vi "filter.hostToFpga.testRunner.vi"(6 "Request.Debug?":bool, 8 "error in":errorcluster, 9 "Watch.List":string[](array[string])=["AAPL"], 10 "Expected OrderBook.Command[]":T1[](array[typedef])=[{"OrderBook Command.Type"=enum."AddOrder", "Side (U8)"=66, "Order Id (U64)"=3544385890602799695, "Quantity (U32)"=20000, "Symbol (U64)"=4702127773838213120, "Price (U64)"=9050, "Executed Quantity (U32)"=0, "Canceled Quantity (U32)"=0, "Remaining Quantity (U32)"=0, "Seconds (U64)"=0, "Nanoseconds (U64)"=0}, {"OrderBook Command.Type"=enum."AddOrder", "Side (U8)"=66, "Order Id (U64)"=3616443484640727631, "Quantity (U32)"=20000, "Symbol (U64)"=4702127773838213120, "Price (U64)"=9050, "Executed Quantity (U32)"=0, "Canceled Quantity (U32)"=0, "Remaining Quantity (U32)"=0, "Seconds (U64)"=0, "Nanoseconds (U64)"=0}, {"OrderBook Command.Type"=enum."AddOrder", "Side (U8)"=66, "Order Id (U64)"=3688501078678655567, "Quantity (U32)"=20000, "Symbol (U64)"=4702127773838213120, "Price (U64)"=9050, "Executed Quantity (U32)"=0, "Canceled Quantity (U32)"=0, "Remaining Quantity (U32)"=0, "Seconds (U64)"=0, "Nanoseconds (U64)"=0}, {"OrderBook Command.Type"=enum."AddOrder", "Side (U8)"=66, "Order Id (U64)"=3760558672716583503, "Quantity (U32)"=20000, "Symbol (U64)"=4702127773838213120, "Price (U64)"=9050, "Executed Quantity (U32)"=0, "Canceled Quantity (U32)"=0, "Remaining Quantity (U32)"=0, "Seconds (U64)"=0, "Nanoseconds (U64)"=0}, {"OrderBook Command.Type"=enum."AddOrder", "Side (U8)"=66, "Order Id (U64)"=3832616266754511439, "Quantity (U32)"=20000, "Symbol (U64)"=4702127773838213120, "Price (U64)"=9050, "Executed Quantity (U32)"=0, "Canceled Quantity (U32)"=0, "Remaining Quantity (U32)"=0, "Seconds (U64)"=0, "Nanoseconds (U64)"=0}, {"OrderBook Command.Type"=enum."AddOrder", "Side (U8)"=66, "Order Id (U64)"=3904673860792439375, "Quantity (U32)"=20000, "Symbol (U64)"=4702127773838213120, "Price (U64)"=9050, "Executed Quantity (U32)"=0, "Canceled Quantity (U32)"=0, "Remaining Quantity (U32)"=0, "Seconds (U64)"=0, "Nanoseconds (U64)"=0}, {"OrderBook Command.Type"=enum."AddOrder", "Side (U8)"=66, "Order Id (U64)"=3976731454830367311, "Quantity (U32)"=20000, "Symbol (U64)"=4702127773838213120, "Price (U64)"=9050, "Executed Quantity (U32)"=0, "Canceled Quantity (U32)"=0, "Remaining Quantity (U32)"=0, "Seconds (U64)"=0, "Nanoseconds (U64)"=0}, {"OrderBook Command.Type"=enum."AddOrder", "Side (U8)"=66, "Order Id (U64)"=4048789048868295247, "Quantity (U32)"=20000, "Symbol (U64)"=4702127773838213120, "Price (U64)"=9050, "Executed Quantity (U32)"=0, "Canceled Quantity (U32)"=0, "Remaining Quantity (U32)"=0, "Seconds (U64)"=0, "Nanoseconds (U64)"=0}, {"OrderBook Command.Type"=enum."AddOrder", "Side (U8)"=66, "Order Id (U64)"=4120846642906223183, "Quantity (U32)"=20000, "Symbol (U64)"=4702127773838213120, "Price (U64)"=9050, "Executed Quantity (U32)"=0, "Canceled Quantity (U32)"=0, "Remaining Quantity (U32)"=0, "Seconds (U64)"=0, "Nanoseconds (U64)"=0}, {"OrderBook Command.Type"=enum."AddOrder", "Side (U8)"=66, "Order Id (U64)"=4697307395209646671, "Quantity (U32)"=20000, "Symbol (U64)"=4702127773838213120, "Price (U64)"=9050, "Executed Quantity (U32)"=0, "Canceled Quantity (U32)"=0, "Remaining Quantity (U32)"=0, "Seconds (U64)"=0, "Nanoseconds (U64)"=0}, {"OrderBook Command.Type"=enum."AddOrder", "Side (U8)"=66, "Order Id (U64)"=4769364989247574607, "Quantity (U32)"=20000, "Symbol (U64)"=4702127773838213120, "Price (U64)"=9050, "Executed Quantity (U32)"=0, "Canceled Quantity (U32)"=0, "Remaining Quantity (U32)"=0, "Seconds (U64)"=0, "Nanoseconds (U64)"=0}] {"Side (U8)" format="%.0x"; "Order Id (U64)" format="%.0x"; "Symbol (U64)" format="%.0x"}, 11 "OrderBook.Commands.in":T1[](array[typedef]) {"Side (U8)" format="%.0x"; "Order Id (U64)" format="%.0x"; "Symbol (U64)" format="%.0x"}) -> (0 "error out":errorcluster={"status"=TRUE, "code"=-61165, "source"="Open FPGA VI Reference in host.bats.parser.tester.vi"}, 1 "Failures.Count":i32, 2 "Passed":bool, 3 "OrderBook.Commands.out":T1[](array[typedef]) {"Side (U8)" format="%.0x"; "Order Id (U64)" format="%.0x"; "Symbol (U64)" format="%.0x"}, 4 "Debug":u64[](array[numeric]) format="%.0x", 5 "GetState":u64[](array[numeric]) format="%.0x")   [LabVIEW 2022 SP3]
uses:
  fpga/common/orderbook.command.ctl
  fpga/common/orderbook.command.type.ctl
  <vilib>/rvi/interface/RandomDataEmulation/nirviRandomDataOpen.vi
  <vilib>/rvi/interface/common/niFpgaCacheSessionInfoDynamic.vi
  <vilib>/Utility/error.llb/Error Cluster From Error Code.vi
  <vilib>/rvi/errors/niLvFpgaAdjustHostInterfaceError.vi
  <vilib>/FPGAPlugInAG/Dynamic/niLvFpga_Close_Dynamic.vi
  <vilib>/rvi/interface/nirviOpenFPGA/nirviOpenFPGA.xnode
  fpga/filter/filter.test.vi
  <vilib>/rvi/interface/nirviReadWriteControl/nirviReadWriteControl.xnode
  <vilib>/rvi/interface/nirviMethod/nirviMethod.xnode
  <vilib>/rvi/interface/nirviCloseFPGA/nirviCloseFPGA.xnode
  <vilib>/rvi/errors/niLvFpgaMergeErrorWithErrorCode.vi
  <vilib>/FPGAPlugInAG/Dynamic/niLvFpga_ReadFifo_Dynamic.vi
  <vilib>/rvi/interface/Simulation/niFpgaSimulationCallBeginRW.vi
  NiFpgaLv.dll
  <vilib>/FPGAPlugInAG/Dynamic/niLvFpga_WriteFifo_Dynamic.vi
panel:
  out "HT-Filter.Commands.In":u64[](array[numeric])=[1, 66, 48, 20000, 4702127773838221344, 9050, 0, 0, 0, 0, 0, 0, 0, 0, 0, 0, 2, 66, 48, 0, 0, 9050, 200, 0, 0, 0, 0, 0, 0, 0, 0, 0, 5, 66, 48, 1400, 6076284164848492576, 9050, 0, 0, 0, 0, 0, 0, 0, 0, 0, 0] format="%.0x"
  out "Failures.Details":bool[][](array[boolean])
  out "Data.size":i32
  in  "Execute?":bool=TRUE
  out "Data":u64[](array[numeric]) format="%.0x"
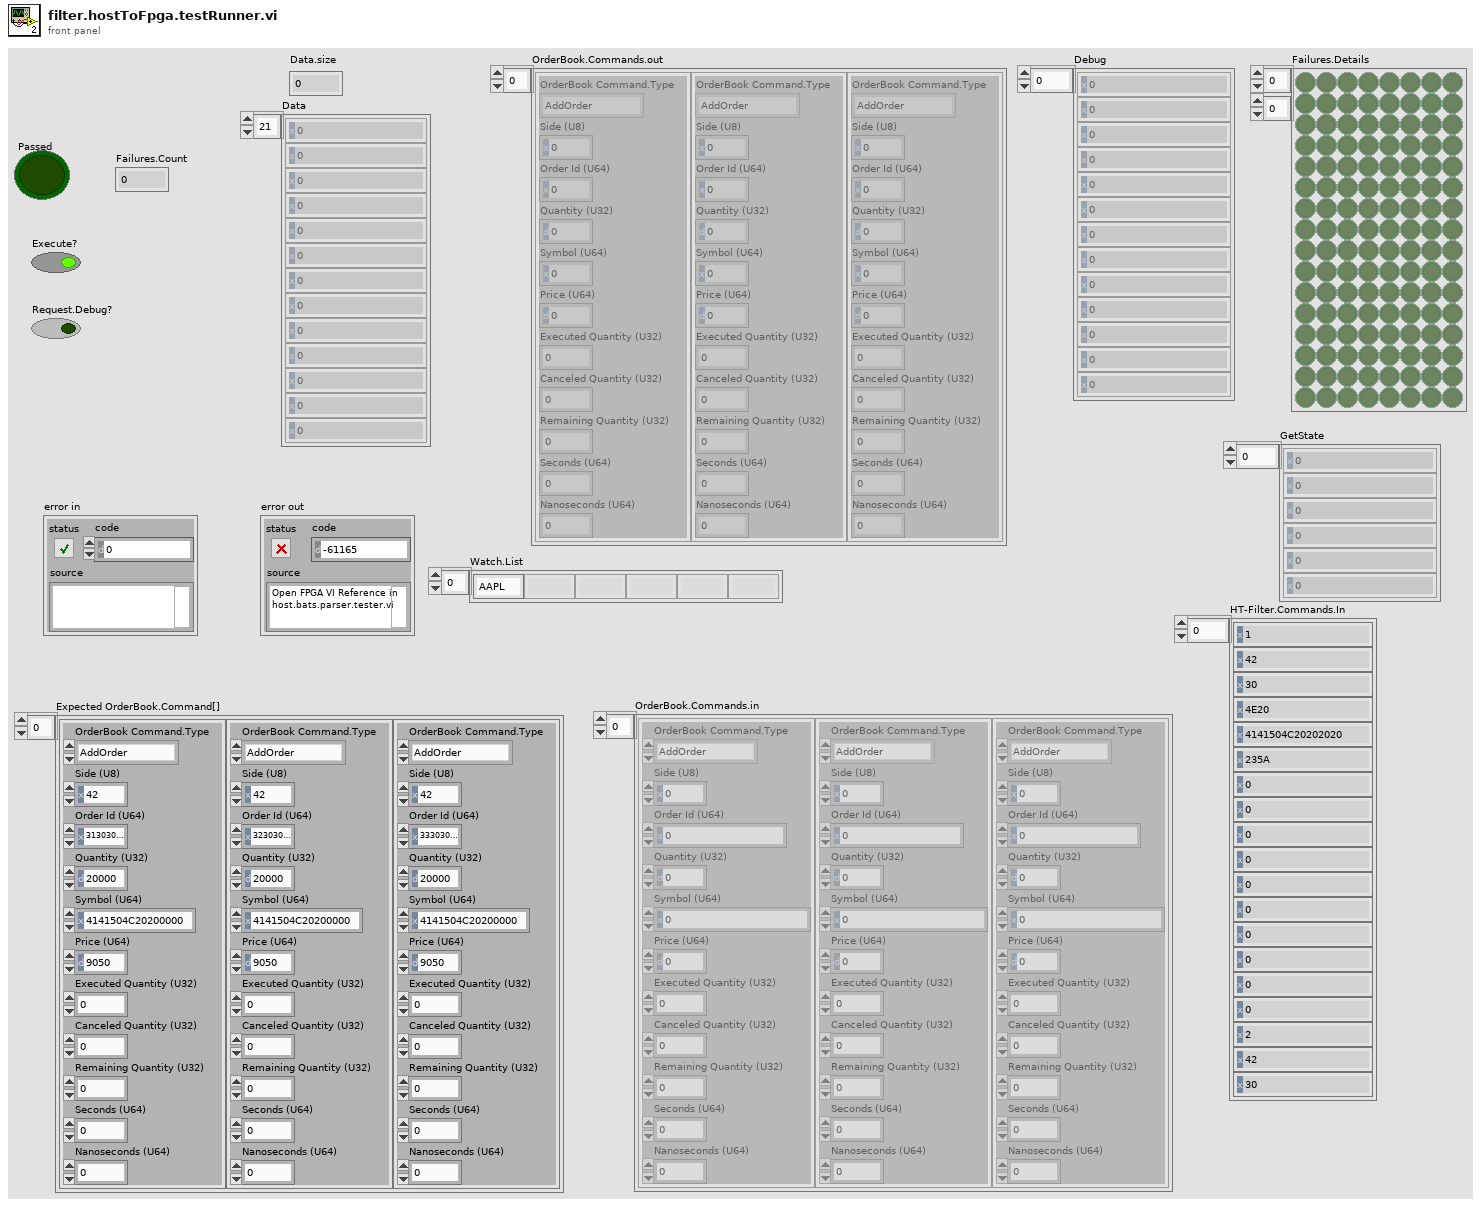
[diagram p1: front panel]
types:
  T1 = typedef "orderbook.command.ctl" = cluster{"OrderBook Command.Type":T2, "Side (U8)":u8, "Order Id (U64)":u64, "Quantity (U32)":u32, "Symbol (U64)":u64, "Price (U64)":u64, "Executed Quantity (U32)":u32, "Canceled Quantity (U32)":u32, "Remaining Quantity (U32)":u32, "Seconds (U64)":u64, "Nanoseconds (U64)":u64}
  T2 = typedef "orderbook.command.type.ctl" = enum16{"Time", "AddOrder", "OrderExecuted", "OrderExecutedAtPrice", "ReduceSize", "ModifyOrder", "DeleteOrder", "Get.State", "Get.All.Orders", "Get.Top"}
  T3 = cluster{"OrderBook Command.Type":bool, "Side (U8)":bool, "Order Id (U64)":bool, "Quantity (U32)":bool, "Symbol (U64)":bool, "Price (U64)":bool, "Executed Quantity (U32)":bool, "Cancelled Quantity (U32)":bool, "Cancelled Quantity (U32) 2":bool, "Executed Quantity (U32) 2":bool, "Cancelled Quantity (U32) 3":bool}
  T4 = cluster{"Index":i32, "x = y?":cluster{"OrderBook Command.Type":bool, "Side (U8)":bool, "Order Id (U64)":bool, "Quantity (U32)":bool, "Symbol (U64)":bool, "Price (U64)":bool, "Executed Quantity (U32)":bool, "Cancelled Quantity (U32)":bool, "Cancelled Quantity (U32) 2":bool, "Executed Quantity (U32) 2":bool, "Cancelled Quantity (U32) 3":bool}}
  T5 = cluster{"Index":i32, "x = y?":cluster{"OrderBook Command.Type":bool, "Side (U8)":bool, "Order Id (U64)":bool, "Quantity (U32)":bool, "Symbol (U64)":bool, "Price (U64)":bool, "Executed Quantity (U32)":bool, "Cancelled Quantity (U32)":bool, "Cancelled Quantity (U32) 2":bool, "Executed Quantity (U32) 2":bool, "Cancelled Quantity (U32) 3":bool}}[]
  T6 = cluster{"OrderBook Command.Type":bool, "Side (U8)":bool, "Order Id (U64)":bool, "Quantity (U32)":bool, "Symbol (U64)":bool, "Price (U64)":bool, "Executed Quantity (U32)":bool, "Canceled Quantity (U32)":bool, "Remaining Quantity (U32)":bool, "Seconds (U64)":bool, "Nanoseconds (U64)":bool}
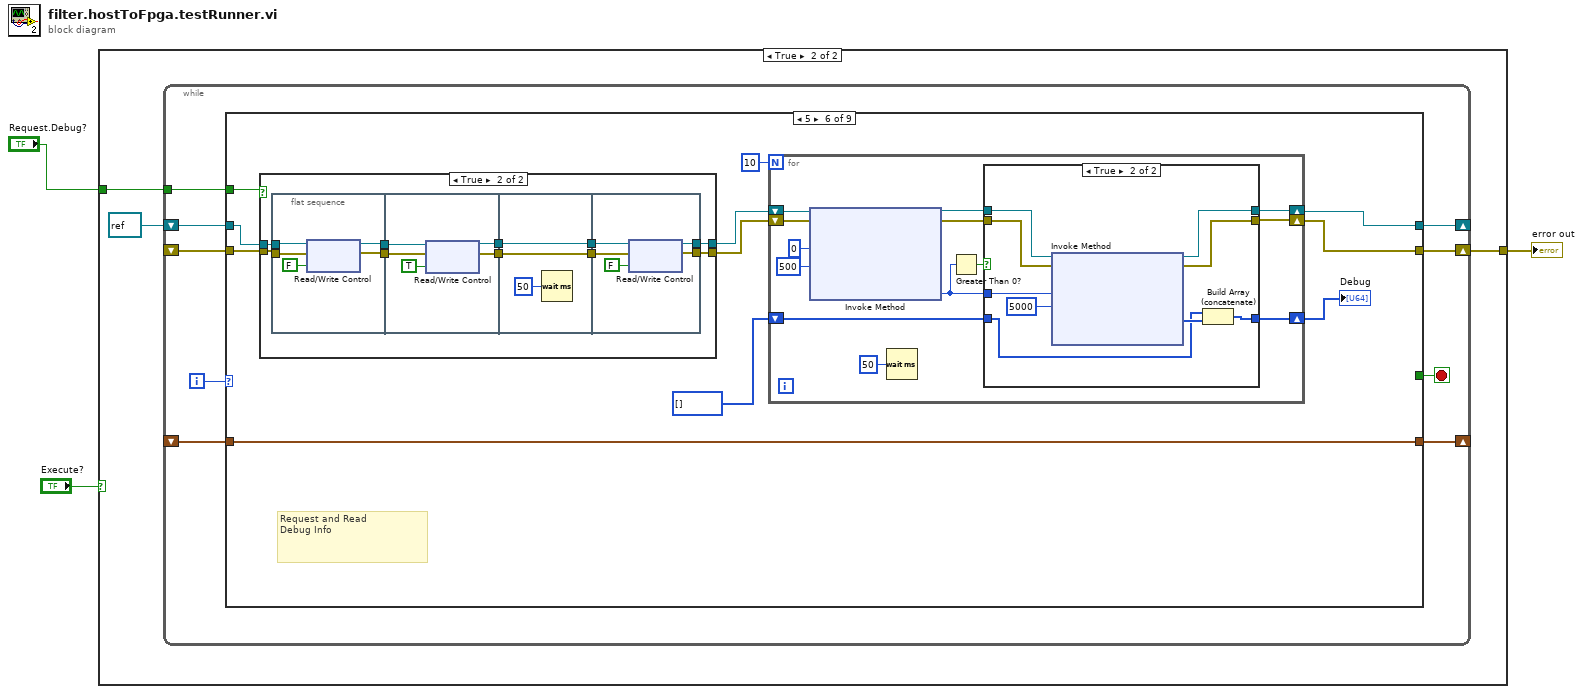
[diagram p0: block diagram]
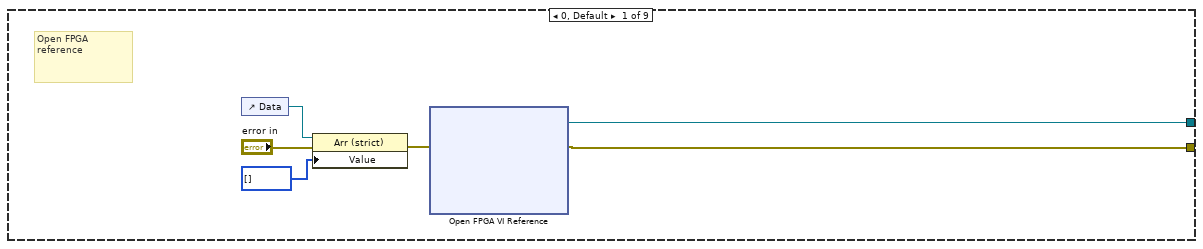
[diagram p3: hidden frame]
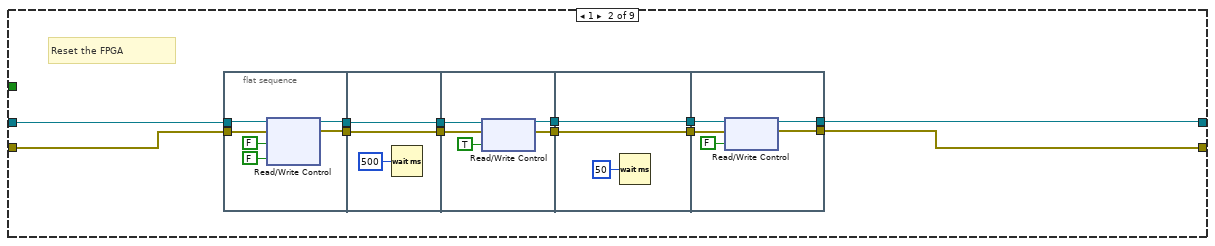
[diagram p4: hidden frame]
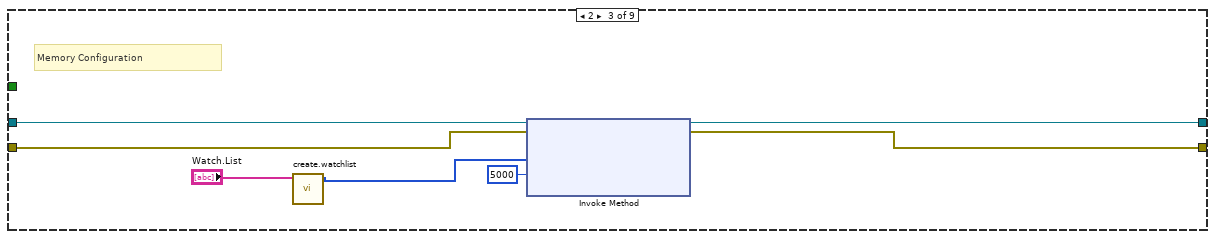
[diagram p5: hidden frame]
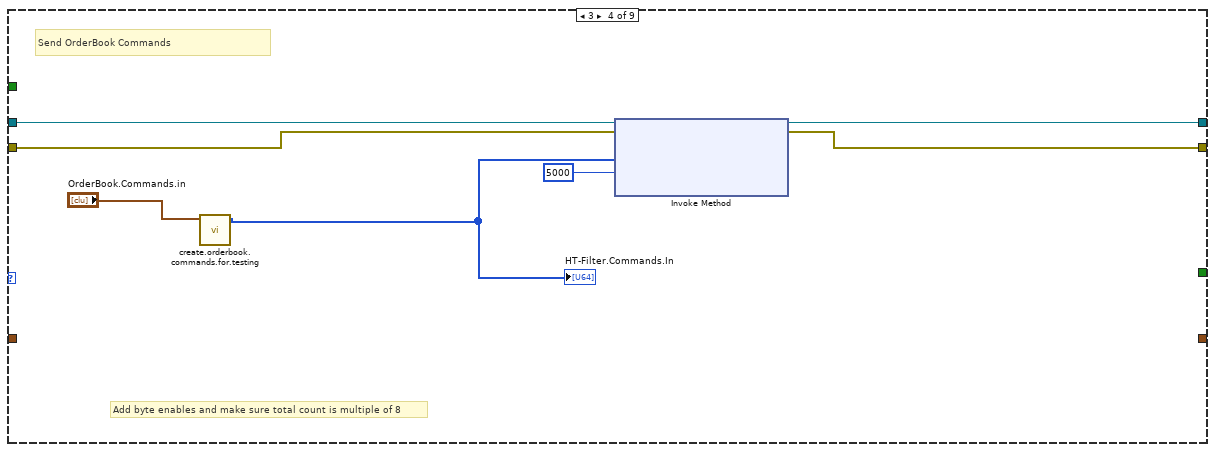
[diagram p6: hidden frame]
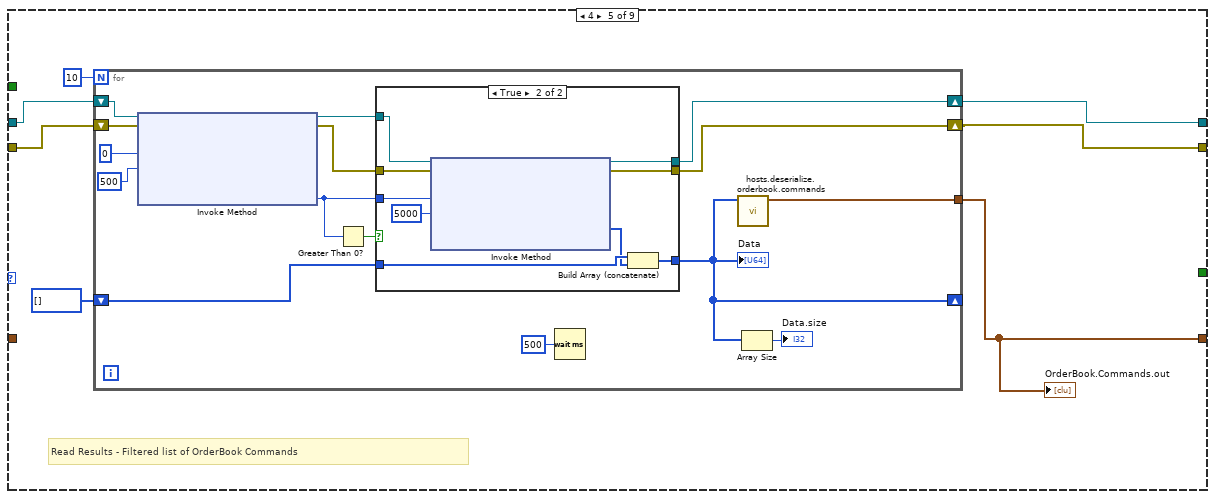
[diagram p7: hidden frame]
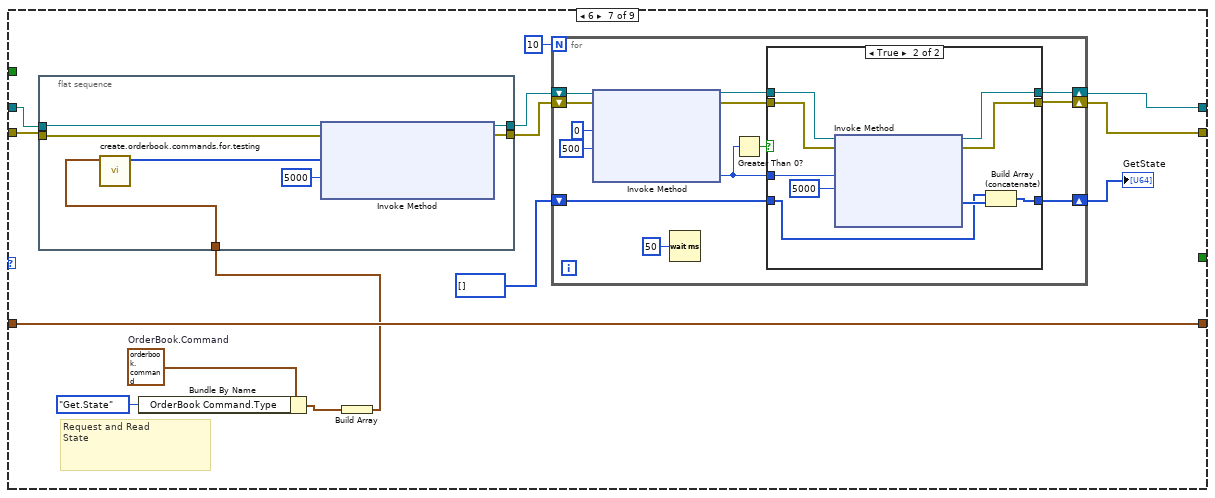
[diagram p11: hidden frame]
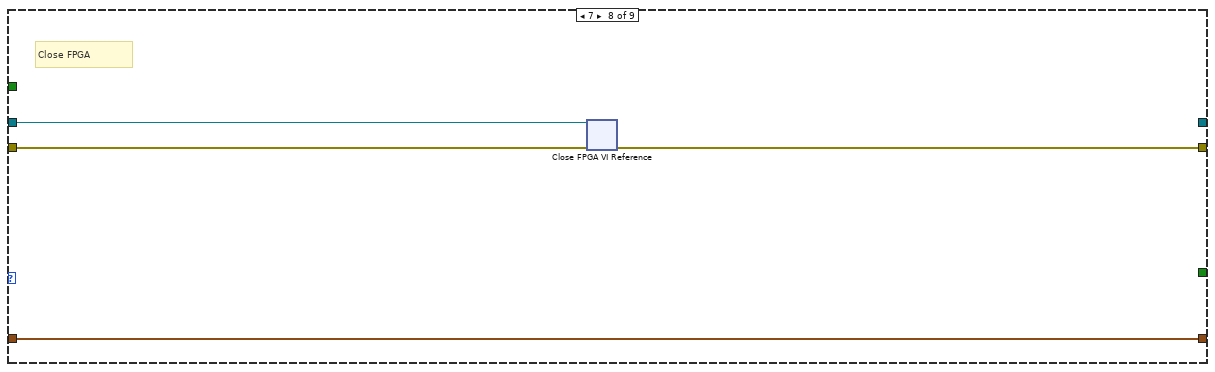
[diagram p13: hidden frame]
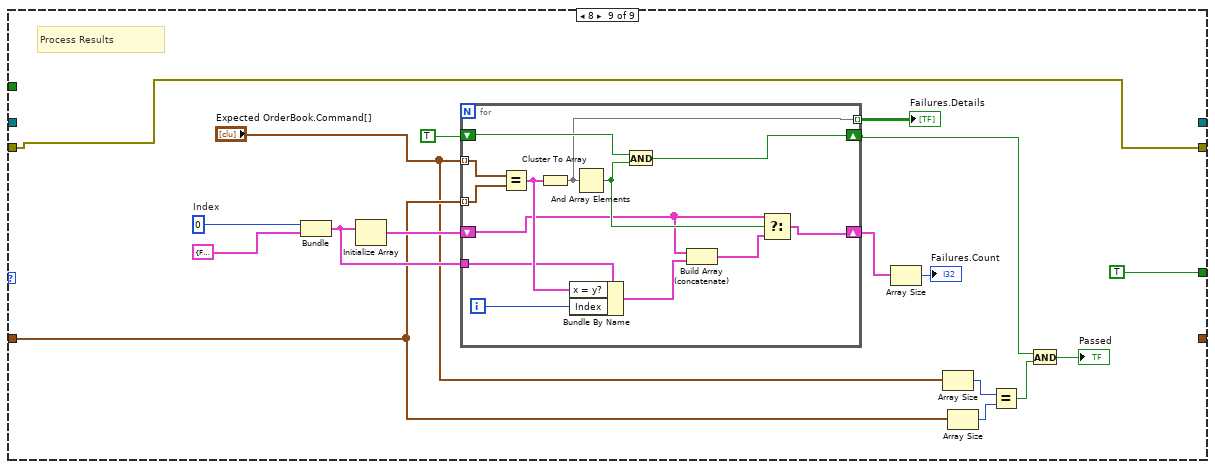
[diagram p14: hidden frame]
diagram:
  n1 = case shown="True" "Execute?" {
    tunnel: [_ w6] -> w3
    tunnel: "Request.Debug?" -> [_ w4]
    frame False {
    }
    frame True {
      n2 = while {
        shift-right: [w13] -> w6
        shift-left: _ -> [w12]
        shift-right: [w11] -> _
        shift-left: _ -> [w10]
        shift-right: [w8] -> _
        shift-left: refnum<k20> refnum ("FPGA VI Reference Out") -> [w9]
        tunnel: w4 -> [w7]
        i -> [w15]
        stop <- w14 stop-if-true
        n3 = case shown="5" w15 {
          tunnel: [_ _ _ _ _ _ _ _ TRUE] -> w14
          tunnel: [w17 w32 w60 w68 w75 w111 w180 w219 w225] -> w13
          tunnel: w12 -> [_ w33 w61 w69 w76 w114 w183 w218 w225]
          tunnel: [_ _ _ _ w74 w107 w176 w217 _] -> w11
          tunnel: w10 -> [_ _ _ _ _ w107 w176 w217 w226]
          tunnel: [w16 w22 w56 w63 w70 w105 w170 _ _] -> w8
          tunnel: w9 -> [_ w23 w57 w64 w71 w106 w171 w216 _]
          tunnel: w7 -> [_ _ _ _ _ w104 _ _ _]
          frame 0, Default {
            # "Open FPGA\nreference"
            n4 = control-ref of="Data"() -> (w19:refnum<vi>)
            n5 = property class="Arr (strict)"(reference=w19, error in="error in", "Value"=u8[] []) -> (error out=w21:errorcluster)  [unwired: 1 out]
            n6 = xnode ("Open FPGA VI Reference")("error in"=w21) -> ("FPGA VI Reference Out"=w16:refnum<k20>, "error out"=w17:errorcluster)  [unwired: 1 in]
          }
          frame 1 {
            # "Reset the FPGA"
            n7 = flat-sequence {
              tunnel: w23 -> [w36]
              tunnel: w33 -> [w37]
              tunnel: [w38] -> w31
              tunnel: [w39] -> w29
              tunnel: w31 -> [w42]
              tunnel: [w42] -> w30
              tunnel: w29 -> [w41]
              tunnel: [w41] -> w28
              tunnel: [w46] -> w25
              tunnel: [w45] -> w27
              tunnel: w30 -> [w44]
              tunnel: w28 -> [w43]
              tunnel: w27 -> [w50]
              tunnel: [w50] -> w26
              tunnel: w25 -> [w49]
              tunnel: [w49] -> w24
              tunnel: [w52] -> w32
              tunnel: [w51] -> w22
              tunnel: w26 -> [w53]
              tunnel: w24 -> [w54]
              frame #0 {
                n8 = xnode "Read/Write Control"("FPGA VI Reference In"=w36, "error in"=w37, "reset"=FALSE, "debug"=FALSE) -> ("FPGA VI Reference Out"=w39:refnum<k20>, "error out"=w38:errorcluster)
              }
              frame #1 {
                n9 = Wait (ms)(milliseconds to wait=u32 500) -> ()  [unwired: 1 out]
              }
              frame #2 {
                n10 = xnode "Read/Write Control"("FPGA VI Reference In"=w43, "error in"=w44, "reset"=TRUE) -> ("FPGA VI Reference Out"=w45:refnum<k20>, "error out"=w46:errorcluster)
              }
              frame #3 {
                n11 = Wait (ms)(milliseconds to wait=u32 50) -> ()  [unwired: 1 out]
              }
              frame #4 {
                n12 = xnode "Read/Write Control"("FPGA VI Reference In"=w53, "error in"=w54, "reset"=FALSE) -> ("FPGA VI Reference Out"=w51:refnum<k20>, "error out"=w52:errorcluster)
              }
            }
          }
          frame 2 {
            # "Memory Configuration"
            n13 = call "create.watchlist.vi"("watch.list"="Watch.List") -> ("memory.config"=w58:u64[])  [unwired: 10 in]
            n14 = xnode "Invoke Method"("FPGA VI Reference In"=w57, "error in"=w61, "Data"=w58, "Timeout (ms)"=5000) -> ("FPGA VI Reference Out"=w56:refnum<k20>, "error out"=w60:errorcluster)  [unwired: 1 out]
          }
          frame 3 {
            # "Add byte enables and make sure total count is multiple of 8"
            # "Send OrderBook Commands"
            n15 = call "create.orderbook.commands.for.testing.vi"("OrderBook.Commands.in"="OrderBook.Commands.in") -> ("Words.Out"=w66:u64[])  [unwired: 10 in]
            "HT-Filter.Commands.In" <- w66
            n16 = xnode "Invoke Method"("FPGA VI Reference In"=w64, "error in"=w69, "Data"=w66, "Timeout (ms)"=5000) -> ("FPGA VI Reference Out"=w63:refnum<k20>, "error out"=w68:errorcluster)  [unwired: 1 out]
          }
          frame 4 {
            # "Read Results - Filtered list of OrderBook Commands"
            n17 = for {
              N: 10 -> [_]
              shift-right: [w79] -> _
              shift-left: u64[] [] -> [w84]
              shift-right: [w83] -> w70
              shift-left: w71 -> [w91]
              shift-right: [w82] -> w75
              shift-left: w76 -> [w90]
              tunnel: [w77] -> w74
              n18 = xnode "Invoke Method"("FPGA VI Reference In"=w91, "error in"=w90, "Number of Elements"=u32 0, "Timeout (ms)"=500) -> ("FPGA VI Reference Out"=w85:refnum<k20>, "error out"=w81:errorcluster, "Elements Remaining"=w86:u32)  [unwired: 1 out]
              n19 = Greater Than 0?(x=w86) -> (x > 0?=w87:bool)
              n20 = case shown="True" w87 {
                tunnel: w86 -> [_ w103]
                tunnel: w85 -> [w93 w101]
                tunnel: [w94 w98] -> w79
                tunnel: w84 -> [w94 w100]
                tunnel: [w93 w97] -> w83
                tunnel: [w92 w96] -> w82
                tunnel: w81 -> [w92 w95]
                frame False {
                }
                frame True {
                  n21 = xnode "Invoke Method"("FPGA VI Reference In"=w101, "error in"=w95, "Number of Elements"=w103, "Timeout (ms)"=5000) -> ("FPGA VI Reference Out"=w97:refnum<k20>, "error out"=w96:errorcluster, "Data"=w99:u64[])  [unwired: 1 out]
                  n22 = Build Array (concatenate)(w100, w99) -> (w98:u64[])
                }
              }
              "Data" <- w79
              n23 = Wait (ms)(milliseconds to wait=u32 500) -> ()  [unwired: 1 out]
              n24 = call "hosts.deserialize.orderbook.commands.vi"("DataIn"=w79) -> ("OrderBook.Command[]"=w77:T1[])  [unwired: 10 in]
              n25 = Array Size(array=w79) -> (size(s)=→"Data.size":i32)
            }
            "OrderBook.Commands.out" <- w74
          }
          frame 5 {
            # "Request and Read\nDebug Info"
            n26 = case shown="True" w104 {
              tunnel: w114 -> [w115 w120]
              tunnel: [w116 w119] -> w113
              tunnel: [w115 w118] -> w112
              tunnel: w106 -> [w116 w117]
              frame False {
              }
              frame True {
                n27 = flat-sequence {
                  tunnel: w117 -> [w128]
                  tunnel: w120 -> [w129]
                  tunnel: [w130] -> w126
                  tunnel: [w131] -> w125
                  tunnel: [w135] -> w124
                  tunnel: [w134] -> w123
                  tunnel: w126 -> [w133]
                  tunnel: w125 -> [w132]
                  tunnel: [w139] -> w122
                  tunnel: w124 -> [w139]
                  tunnel: w123 -> [w138]
                  tunnel: [w138] -> w121
                  tunnel: w122 -> [w143]
                  tunnel: w121 -> [w142]
                  tunnel: [w141] -> w118
                  tunnel: [w140] -> w119
                  frame #0 {
                    n28 = xnode "Read/Write Control"("FPGA VI Reference In"=w128, "error in"=w129, "debug"=FALSE ("reset")) -> ("FPGA VI Reference Out"=w131:refnum<k20>, "error out"=w130:errorcluster)
                  }
                  frame #1 {
                    n29 = xnode "Read/Write Control"("FPGA VI Reference In"=w132, "error in"=w133, "debug"=TRUE ("reset")) -> ("FPGA VI Reference Out"=w134:refnum<k20>, "error out"=w135:errorcluster)
                  }
                  frame #2 {
                    n30 = Wait (ms)(milliseconds to wait=u32 50) -> ()  [unwired: 1 out]
                  }
                  frame #3 {
                    n31 = xnode "Read/Write Control"("FPGA VI Reference In"=w142, "error in"=w143, "debug"=FALSE ("reset")) -> ("FPGA VI Reference Out"=w140:refnum<k20>, "error out"=w141:errorcluster)
                  }
                }
              }
            }
            n32 = for {
              N: 10 -> [_]
              shift-right: [w151] -> w105
              shift-left: w113 -> [w157]
              shift-right: [w150] -> w111
              shift-left: w112 -> [w156]
              shift-right: [w152] -> w110
              shift-left: u64[] [] -> [w146]
              n33 = xnode "Invoke Method"("FPGA VI Reference In"=w157, "error in"=w156, "Number of Elements"=u32 0, "Timeout (ms)"=500) -> ("FPGA VI Reference Out"=w149:refnum<k20>, "error out"=w148:errorcluster, "Elements Remaining"=w147:u32)  [unwired: 1 out]
              n34 = Wait (ms)(milliseconds to wait=u32 50) -> ()  [unwired: 1 out]
              n35 = Greater Than 0?(x=w147) -> (x > 0?=w153:bool)
              n36 = case shown="True" w153 {
                tunnel: [w158 w168] -> w152
                tunnel: [w160 w167] -> w151
                tunnel: [w159 w166] -> w150
                tunnel: w149 -> [w160 w165]
                tunnel: w148 -> [w159 w164]
                tunnel: w147 -> [_ w163]
                tunnel: w146 -> [w158 w161]
                frame False {
                }
                frame True {
                  n37 = xnode "Invoke Method"("FPGA VI Reference In"=w165, "error in"=w164, "Number of Elements"=w163, "Timeout (ms)"=5000) -> ("FPGA VI Reference Out"=w167:refnum<k20>, "error out"=w166:errorcluster, "Data"=w169:u64[])  [unwired: 1 out]
                  n38 = Build Array (concatenate)(w161, w169) -> (w168:u64[])
                }
              }
            }
            "Debug" <- w110
          }
          frame 6 {
            w175 = T1 {"OrderBook Command.Type"=enum."AddOrder", "Side (U8)"=66, "Order Id (U64)"=48, "Quantity (U32)"=20000, "Symbol (U64)"=4702127773838221344, "Price (U64)"=9050, "Executed Quantity (U32)"=0, "Canceled Quantity (U32)"=0, "Remaining Quantity (U32)"=0, "Seconds (U64)"=0, "Nanoseconds (U64)"=0}  # OrderBook.Command
            # "Request and Read\nState"
            n39 = flat-sequence {
              tunnel: [w188] -> w181
              tunnel: [w187] -> w182
              tunnel: w171 -> [w189]
              tunnel: w183 -> [w190]
              tunnel: w172 -> [w184]
              frame #0 {
                n40 = call "create.orderbook.commands.for.testing.vi"("OrderBook.Commands.in"=w184) -> ("Words.Out"=w185:u64[])  [unwired: 10 in]
                n41 = xnode "Invoke Method"("FPGA VI Reference In"=w189, "error in"=w190, "Data"=w185, "Timeout (ms)"=5000) -> ("FPGA VI Reference Out"=w187:refnum<k20>, "error out"=w188:errorcluster)  [unwired: 1 out]
              }
            }
            n42 = Bundle By Name(cluster=w175, "OrderBook Command.Type"=orderbook.command.type."Get.State") -> (w173:T1)
            n43 = Build Array(w173) -> (w172:T1[])
            n44 = for {
              N: 10 -> [_]
              shift-right: [w197] -> w170
              shift-left: w182 -> [w203]
              shift-right: [w196] -> w180
              shift-left: w181 -> [w202]
              shift-right: [w198] -> w179
              shift-left: u64[] [] -> [w192]
              n45 = xnode "Invoke Method"("FPGA VI Reference In"=w203, "error in"=w202, "Number of Elements"=u32 0, "Timeout (ms)"=500) -> ("FPGA VI Reference Out"=w195:refnum<k20>, "error out"=w194:errorcluster, "Elements Remaining"=w193:u32)  [unwired: 1 out]
              n46 = Wait (ms)(milliseconds to wait=u32 50) -> ()  [unwired: 1 out]
              n47 = Greater Than 0?(x=w193) -> (x > 0?=w199:bool)
              n48 = case shown="True" w199 {
                tunnel: [w204 w214] -> w198
                tunnel: [w206 w213] -> w197
                tunnel: [w205 w212] -> w196
                tunnel: w195 -> [w206 w211]
                tunnel: w194 -> [w205 w210]
                tunnel: w193 -> [_ w209]
                tunnel: w192 -> [w204 w207]
                frame False {
                }
                frame True {
                  n49 = xnode "Invoke Method"("FPGA VI Reference In"=w211, "error in"=w210, "Number of Elements"=w209, "Timeout (ms)"=5000) -> ("FPGA VI Reference Out"=w213:refnum<k20>, "error out"=w212:errorcluster, "Data"=w215:u64[])  [unwired: 1 out]
                  n50 = Build Array (concatenate)(w207, w215) -> (w214:u64[])
                }
              }
            }
            "GetState" <- w179
          }
          frame 7 {
            # "Close FPGA"
            n51 = xnode "Close FPGA VI Reference"("FPGA VI Reference In"=w216, "error in"=w218) -> ("error out"=w219:errorcluster)
          }
          frame 8 {
            w229 = 0  # Index
            # "Process Results"
            n52 = Bundle("Index"=w229, "x = y?"=T3 {"OrderBook Command.Type"=FALSE, "Side (U8)"=FALSE, "Order Id (U64)"=FALSE, "Quantity (U32)"=FALSE, "Symbol (U64)"=FALSE, "Price (U64)"=FALSE, "Executed Quantity (U32)"=FALSE, "Cancelled Quantity (U32)"=FALSE, "Cancelled Quantity (U32) 2"=FALSE, "Executed Quantity (U32) 2"=FALSE, "Cancelled Quantity (U32) 3"=FALSE}) -> (w231:T4)  [unwired: 1 in]
            n53 = Initialize Array(w231) -> (w230:T5)  [unwired: 1 in]
            n54 = for {
              tunnel: "Expected OrderBook.Command[]" -> [w249] mode=indexing
              tunnel: w226 -> [w248] mode=indexing
              shift-right: [w246] -> w235
              shift-left: TRUE -> [w247]
              shift-right: [w244] -> w232
              shift-left: w230 -> [w239]
              tunnel: w231 -> [w242]
              tunnel: [w237] -> w220 mode=indexing
              i -> [w241]
              n55 = Equal?(x=w249, y=w248) -> (x = y?=w243:T6)
              n56 = Cluster To Array(cluster=w243) -> (array=w237:bool[])
              n57 = Bundle By Name(cluster=w242, "x = y?"=w243, "Index"=w241) -> (w240:T4)
              n58 = And Array Elements(Boolean array=w237) -> (logical AND=w245:bool)
              n59 = And(x=w247, y=w245) -> (x .and. y?=w246:bool)
              n60 = Build Array (concatenate)(w239, w240) -> (w238:T5)
              n61 = Select(t=w239, s=w245, f=w238) -> (s? t:f=w244:T5)
            }
            "Failures.Details" <- w220
            n62 = Array Size(array=w232) -> (size(s)=→"Failures.Count":i32)
            n63 = Array Size(array="Expected OrderBook.Command[]") -> (size(s)=w223:i32)
            n64 = Array Size(array=w226) -> (size(s)=w222:i32)
            n65 = Equal?(x=w223, y=w222) -> (x = y?=w221:bool)
            n66 = And(x=w235, y=w221) -> (x .and. y?=→"Passed":bool)
          }
        }
      }
    }
  }
  "error out" <- w3
